vi "playInactivitySound.vi"(11 "sounds":T1={"welcome sound"=path "C:/Users/wingX/Documents/WingXSVN/labview/daq test/sounds/welcome.wav", "play welcome"=TRUE, "got fly sound"=path "C:/Users/wingX/Documents/WingXSVN/labview/daq test/sounds/gotafly.wav", "play got fly"=FALSE, "discard sound"=path "C:/Users/wingX/Documents/WingXSVN/labview/daq test/sounds/blowingback.wav", "play discard"=FALSE, "finish sound"=path "C:/Users/wingX/Documents/WingXSVN/labview/daq test/sounds/finishedmeasuring.wav", "play finish"=TRUE, "inactivity alarm sound"=path "C:/Users/wingX/Documents/WingXSVN/labview/daq test/sounds/finishedmeasuring.wav", "play inactivity\nalarm"=TRUE}) -> ()   [LabVIEW 2012]
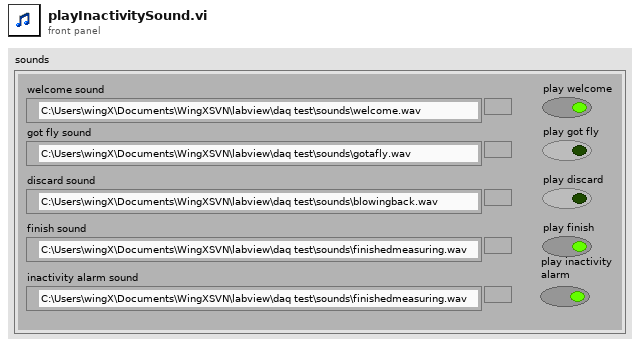
[diagram p1: front panel]
types:
  T1 = cluster{"welcome sound":path, "play welcome":bool, "got fly sound":path, "play got fly":bool, "discard sound":path, "play discard":bool, "finish sound":path, "play finish":bool, "inactivity alarm sound":path, "play inactivity\nalarm":bool}
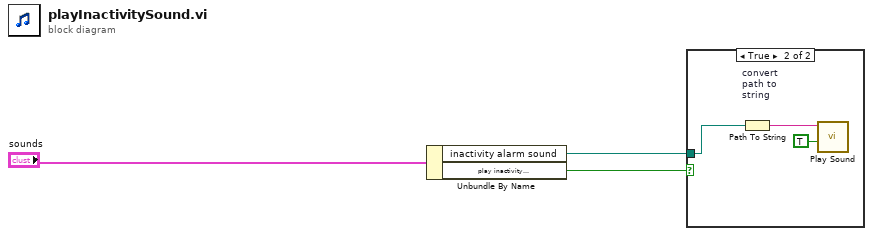
[diagram p0: block diagram]
diagram:
  n1 = Unbundle By Name("sounds") -> ("inactivity alarm sound"=w3:path, "play inactivity\nalarm"=w1:bool)
  n2 = case shown="True" w1 {
    tunnel: w3 -> [_ w5]
    frame False {
    }
    frame True {
      n3 = Path To String "convert\npath to\nstring"(path=w5) -> (string=w6:string)
      n4 = call "Play Sound.vi"("Asynchronous? (F)"=TRUE, "Sound Name"=w6) -> ()  [unwired: 3 in, 1 out]
    }
  }
